vi "Poisson Randomize Array.vi"(11 "Array":dbl[](array[numeric])) -> (3 "Poisson Randomized Array":dbl[](array[numeric]))   [LabVIEW 2019]
uses:
  <vilib>/gmath/NI_Gmath.lvlib
panel:
  out "Error Out":errorcluster
  in  "Error In":errorcluster
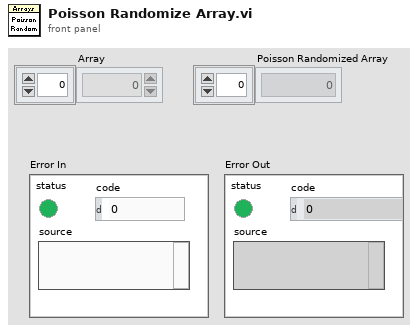
[diagram p1: front panel]
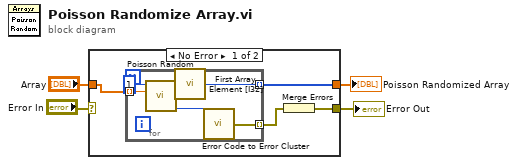
[diagram p0: block diagram]
diagram:
  n1 = case shown="No Error" "Error In" {
    selector: "Error In" -> [_ w16]
    tunnel: [w8 w15] -> w4
    tunnel: "Array" -> [w7 w15]
    tunnel: [w5 w16] -> w1
    frame No Error {
      n2 = for {
        tunnel: w7 -> [w14] mode=indexing
        tunnel: [w11] -> w8 mode=indexing
        tunnel: [w9] -> w6 mode=indexing
        n3 = call <vilib>:"Poisson Random.vi"("lambda"=w14, "samples"=1) -> ("error"=w10:i32, "Poisson random data"=w12:i32[])  [unwired: 8 in]
        n4 = call "First Array Element [I32].vi"("Array"=w12) -> ("First Element"=w11:i32)  [unwired: 8 in]
        n5 = call "Error Code to Error Cluster.vi"("Error Code"=w10) -> ("Error Out"=w9:errorcluster)  [unwired: 14 in]
      }
      n6 = Merge Errors(w6) -> (w5:errorcluster)
    }
    frame Error {
    }
  }
  "Poisson Randomized Array" <- w4
  "Error Out" <- w1
